vi "Wait on Async ACQ Notification.vi"(8 "error in (no error)":errorcluster, 9 "timeout in ms (-1)":i32, 11 "Async ACQ Notifier in":refnum<notifier>) -> (0 "error out":errorcluster, 1 "timed out?":bool, 2 "Async ACQ":T1, 3 "Async ACQ Notifier out":refnum<notifier>)   [LabVIEW 2014, in "WINFAS 2 Data Queue.lvlib"]
uses:
  WINFAS 2 Data Queue.lvlib
  Async Acquisition Data Cluster.ctl
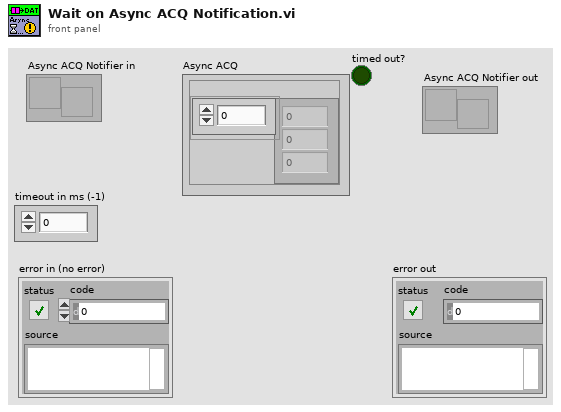
[diagram p1: front panel]
types:
  T1 = typedef "WINFAS 2 Data Queue.lvlib/Async Acquisition Data Cluster.ctl" = cluster{"Data":sgl[]}
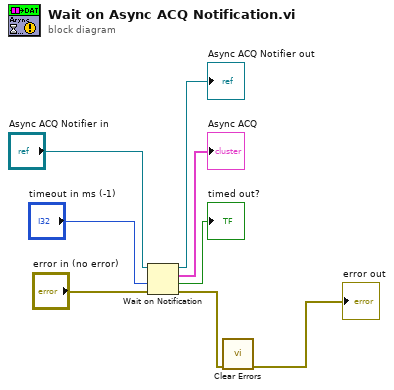
[diagram p0: block diagram]
diagram:
  n1 = Wait on Notification(notifier="Async ACQ Notifier in", timeout in ms (-1)="timeout in ms (-1)", error in (no error)="error in (no error)") -> (notifier out=→"Async ACQ Notifier out":refnum<notifier>, notification=→"Async ACQ":T1, timed out?=→"timed out?":bool, error out=w2:errorcluster)  [unwired: 1 in]
  n2 = call <vilib>:"Clear Errors.vi"("error in (no error)"=w2) -> ("error out"=→"error out":errorcluster)  [unwired: 5 in, 1 out]
